vi "Stitching-Column selection window.vi"() -> (1 "Cancelled":bool, 2 "Base directory":path, 3 "Column index":i32)   [LabVIEW 2013]
uses:
  <vilib>/Utility/miscctls.llb/LVPointTypeDef.ctl
  Global Variables/General Globals.vi
panel:
  in  "Base directory":path
  in  "Cancel":bool
  in  "OK":bool
  in  "Selector":u16(ring)=3 items=["X", "Y", "Z", "Name", "Folders", "6", "7", "8", "9", "10", "11", "12"]
  # "Select the column holding the names of the dataset folders you want to generate the collage from."
  # "Tip 1: If the column is unnamed right click on it and use the \"Edit column name\" option to name it before you can select it in this window.\nTip 2: It is possible to select specific rows using the Ctrl and/or the Shift key on the keyboard before generating a collage."
  # "Select the Base directory containing the dataset folders you want to generate the collage from."
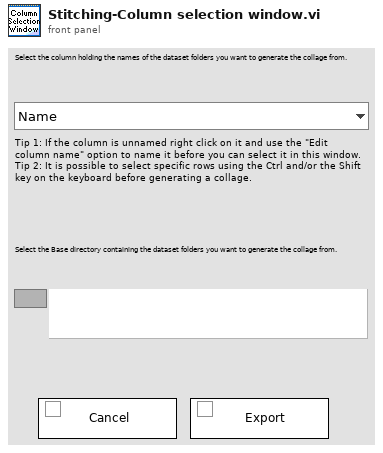
[diagram p1: front panel]
types:
  T1 = typedef "LVPointTypeDef.ctl" = cluster{"Horizontal":i16, "Vertical":i16}
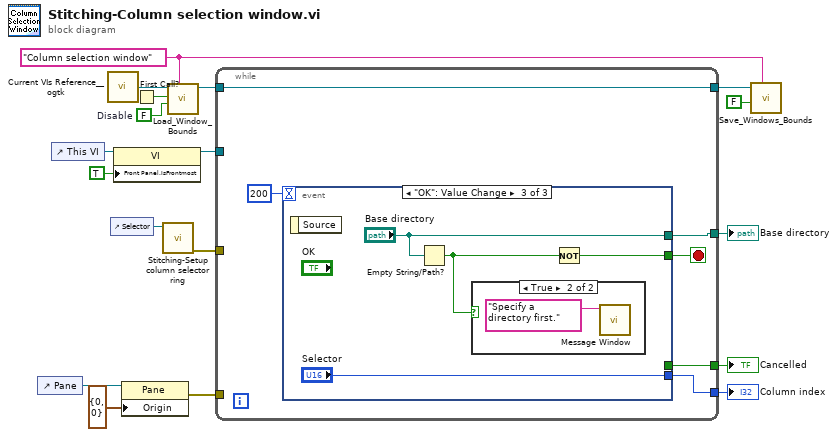
[diagram p0: block diagram]
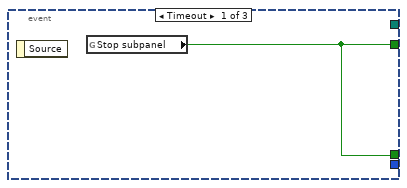
[diagram p2: hidden frame]
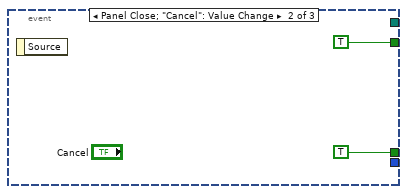
[diagram p3: hidden frame]
diagram:
  w9 = FALSE  # Disable
  w8 = "Column selection window" ("Window Name (i.e. Key)")
  n1 = control-ref of="Pane"() -> (w13:refnum<vi>)
  n2 = control-ref of="This VI"() -> (w17:refnum<vi>)
  n3 = call "Current VIs Reference__ogtk.vi"() -> ("Current VI's reference"=w11:refnum<vi>)  [unwired: 5 in]
  n4 = control-ref of="Selector"() -> (w1:refnum<vi>)
  n5 = property on="Property Node" class="VI"(reference=w17, "Front Panel.IsFrontmost"=TRUE ("Front Panel Window:Is Frontmost")) -> (reference out=w16:refnum<vi>)  [unwired: 1 in, 1 out]
  n6 = property class="Pane"(reference=w13, "Origin"=T1 {"Horizontal"=0, "Vertical"=0}) -> (error out=w14:errorcluster)  [unwired: 1 in, 1 out]
  n7 = First Call?() -> (First Call?: T/F=w10:bool)
  n8 = call "Stitching-Setup column selector ring.vi"("Ring in"=w1) -> ("error out"=w4:errorcluster)  [unwired: 10 in]
  n9 = call "Load_Window_Bounds.vi"("Window Name (i.e. Key)"=w8, "Disable"=w9, "First Call"=w10, "Window VI's Ref"=w11) -> ("reference out"=w6:refnum<vi>)  [unwired: 4 in, 3 out]
  n10 = while {
    tunnel: w14 -> [_]
    tunnel: w16 -> [_]
    tunnel: [w22] -> w12
    tunnel: w6 -> [w21]
    tunnel: [w21] -> w5
    tunnel: w4 -> [_]
    tunnel: [w20] -> w3
    tunnel: [w19] -> w2
    stop <- w24 stop-if-true
    n11 = event shown="[2] \"OK\": Value Change" {
      selector: _ -> [_ _ _]
      dyn-events: _ -> [_ _ _]
      timeout: 200 -> [_ _ _]
      tunnel: [w25 TRUE ("Stop?") w29] -> w24
      tunnel: [w25 TRUE ("Stop subpanel") _] -> w22
      tunnel: [_ _ "Selector"] -> w20
      tunnel: [_ _ "Base directory"] -> w19
      event Timeout {
        n12 = event-data() -> ()  [unwired: 1 in, 1 out]
        n13 = global read "General Globals.vi" "Stop subpanel"() -> (w25:bool)
      }
      event Panel Close; "Cancel": Value Change {
        n14 = event-data() -> ()  [unwired: 1 in, 1 out]
      }
      event "OK": Value Change {
        n15 = event-data() -> ()  [unwired: 1 in, 1 out]
        n16 = Empty String/Path?(string/path="Base directory") -> (empty?=w28:bool)
        n17 = case shown="True" w28 {
          frame False {
          }
          frame True {
            n18 = call "Message Window.vi"("Message string"="Specify a directory first.") -> ()  [unwired: 10 in, 1 out]
          }
        }
        n19 = Not(x=w28) -> (.not. x?=w29:bool)
      }
    }
  }
  "Cancelled" <- w12
  "Column index" <- w3
  "Base directory" <- w2
  n20 = call "Save_Windows_Bounds.vi"("Window Name (i.e. Key)"=w8, "Front Panel Window:Open"=FALSE, "Window VI's Ref"=w5) -> ()  [unwired: 8 in, 1 out]
